vi "ConsumeCoord.vi"(8 "error in (no error)":errorcluster, 11 "PathTokenizer in":refnum<class "PathTokenizer.lvclass">) -> (0 "error out":errorcluster, 3 "PathTokenizer out":refnum<class "PathTokenizer.lvclass">)   [LabVIEW 2019, in "PathTokenizer.lvclass"]
uses:
  PathTokenizer.lvclass
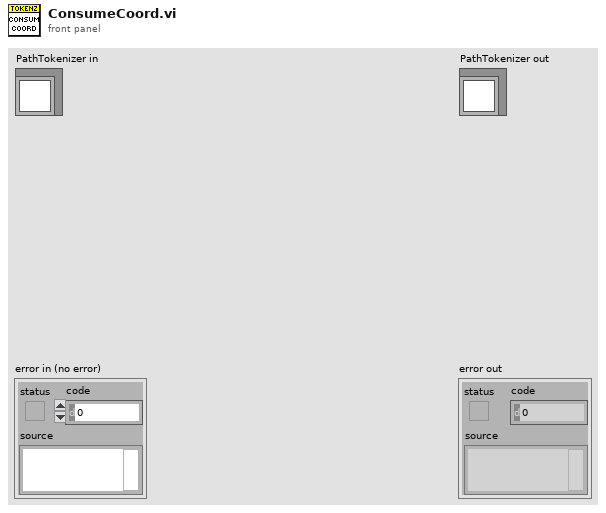
[diagram p1: front panel]
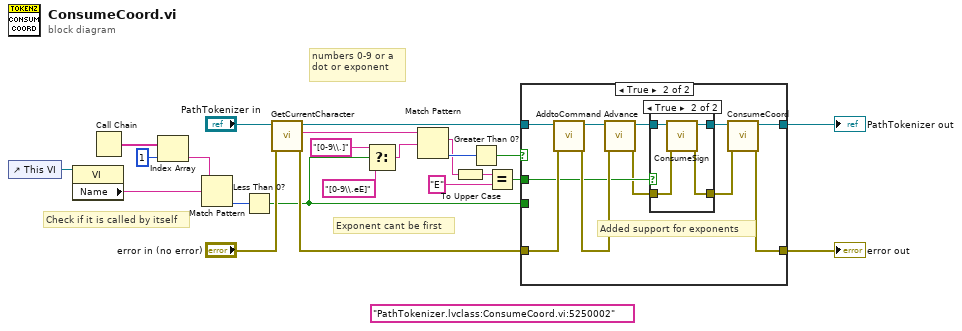
[diagram p0: block diagram]
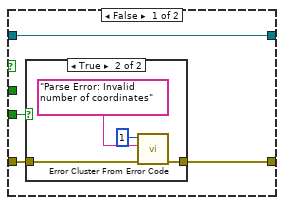
[diagram p2: hidden frame]
diagram:
  (unwired) "PathTokenizer.lvclass:ConsumeCoord.vi:5250002"
  # "Check if it is called by itself"
  # "Exponent cant be first"
  # "numbers 0-9 or a dot or exponent"
  n1 = control-ref of="This VI"() -> (w7:refnum<vi>)
  n2 = property class="VI"(reference=w7) -> ("Name"=w3:string)  [unwired: 1 in, 2 out]
  n3 = Call Chain() -> (call chain=w5:string[])
  n4 = Index Array(array=w5, index=1) -> (element=w4:string)
  n5 = Match Pattern(string=w4, regular expression=w3) -> (offset past match=w2:i32)  [unwired: 1 in, 3 out]
  n6 = Less Than 0?(x=w2) -> (x < 0?=w1:bool)
  n7 = call "GetCurrentCharacter.vi"("error in (no error)"="error in (no error)", "PathTokenizer in"="PathTokenizer in") -> ("error out"=w16:errorcluster, "Current Character"=w21:string, "PathTokenizer out"=w19:refnum<class "PathTokenizer.lvclass">)  [unwired: 7 in]
  n8 = Select(t="[0-9\\.]", s=w1, f="[0-9\\.eE]" ("regular expression")) -> (s? t:f=w10:string)
  n9 = Match Pattern(string=w21, regular expression=w10) -> (match substring=w14:string, offset past match=w20:i32)  [unwired: 1 in, 2 out]
  n10 = To Upper Case(1:w14) -> (0:w12:string)
  n11 = Greater Than 0?(x=w20) -> (x > 0?=w17:bool)
  n12 = Equal?(x=w12, y="E") -> (x = y?=w11:bool)
  n13 = case shown="True" w17 {
    tunnel: w19 -> [w27 w43]
    tunnel: [w27 w40] -> w18
    tunnel: w16 -> [w25 w42]
    tunnel: [w26 w38] -> w15
    tunnel: w1 -> [w24 _]
    tunnel: w11 -> [_ w35]
    frame False {
      n14 = case shown="True" w24 {
        tunnel: [w28 w32] -> w26
        tunnel: w25 -> [w28 w31]
        frame False {
        }
        frame True {
          n15 = call <vilib>:"Error Cluster From Error Code.vi"("error in (no error)"=w31, "error message (\"\")"="Parse Error: Invalid number of coordinates" ("error message (\"\")"), "error code (0)"=1) -> ("error out"=w32:errorcluster)  [unwired: 6 in]
        }
      }
    }
    frame True {
      # "Added support for exponents"
      n16 = call "AddtoCommand.vi"("error in (no error)"=w42, "PathTokenizer in"=w43) -> ("error out"=w39:errorcluster, "PathTokenizer out"=w41:refnum<class "PathTokenizer.lvclass">)  [unwired: 8 in]
      n17 = call "Advance.vi"("error in (no error)"=w39, "PathTokenizer in"=w41) -> ("error out"=w34:errorcluster, "PathTokenizer out"=w37:refnum<class "PathTokenizer.lvclass">)  [unwired: 8 in]
      n18 = case shown="True" w35 {
        tunnel: w37 -> [w45 w49]
        tunnel: [w45 w48] -> w36
        tunnel: w34 -> [w44 w47]
        tunnel: [w44 w46] -> w33
        frame False {
        }
        frame True {
          n19 = call "ConsumeSign.vi"("error in (no error)"=w47, "PathTokenizer in"=w49) -> ("error out"=w46:errorcluster, "PathTokenizer out"=w48:refnum<class "PathTokenizer.lvclass">)  [unwired: 8 in]
        }
      }
      n20 = call "ConsumeCoord.vi"("error in (no error)"=w33, "PathTokenizer in"=w36) -> ("error out"=w38:errorcluster, "PathTokenizer out"=w40:refnum<class "PathTokenizer.lvclass">)  [unwired: 8 in]
    }
  }
  "error out" <- w15
  "PathTokenizer out" <- w18
